vi "FazerGolPelaLateral.vi"(9 "balls":T7[](array[typedef]), 10 "Robot in":T1, 11 "IA State":T6={"our_robots"=[], "enemy_robots"=[], "balls"=[], "geometry"={"field_length"=0, "field_width"=0, "goal_width"=0, "goal_depth"=0, "center_circle_radius"=0, "defense_width"=0, "defense_depth"=0, "free_kick_from_defense_dist"=0, "penalty_spot_from_field_line_dist"=0, "penalty_line_from_spot_dist"=0, "half_moon_depth"=0, "half_moon_width"=0}, "IA Judge"={"stage"="", "command"="", "our_goalie_id"=0.0, "enemy_goalie_id"=0.0, "command enum"=enum."Halt", "Time"=enum."Azul"}, "Received Timestamp"=timestamp(0 s since 1904-01-01), "Events"={"Touch"=FALSE, "id touch"=0.0, "Ball out of \nVision"=FALSE, "Ball inside \nGoalie area"=FALSE, "Robot not responding"=FALSE, "Robots responding status"=[1.0, 1.0, 1.0, 1.0, 1.0, 1.0], "Enemy Ball \nPossession"=FALSE, "Id ini Possession"=0.0, "Ball Possesion"=FALSE, "Id Possesion"=0.0, "Ball at\nour goal side"=FALSE, "Ball at\ntouchline"=FALSE, "Ball at\nenemy goal side"=FALSE}}) -> (3 "Cluster de saída":T1)   [LabVIEW 2018]
doc: "Função que lida com o atacante quando em \"Fazer gol pela lateral\"."
uses:
  Core/AI Robot.ctl
  Intel/Functions Enum.ctl
  Intel/AttackerStates.ctl
  Path Planning/RRT/PathDests.ctl
  Path Planning/RRT/PathDest.ctl
  Core/AI Ball.ctl
  Core/AI Input.ctl
  Core/Field Size.ctl
  Core/AI Judge.ctl
  Intel/Command Enum.ctl
  Util/Events/Events.ctl
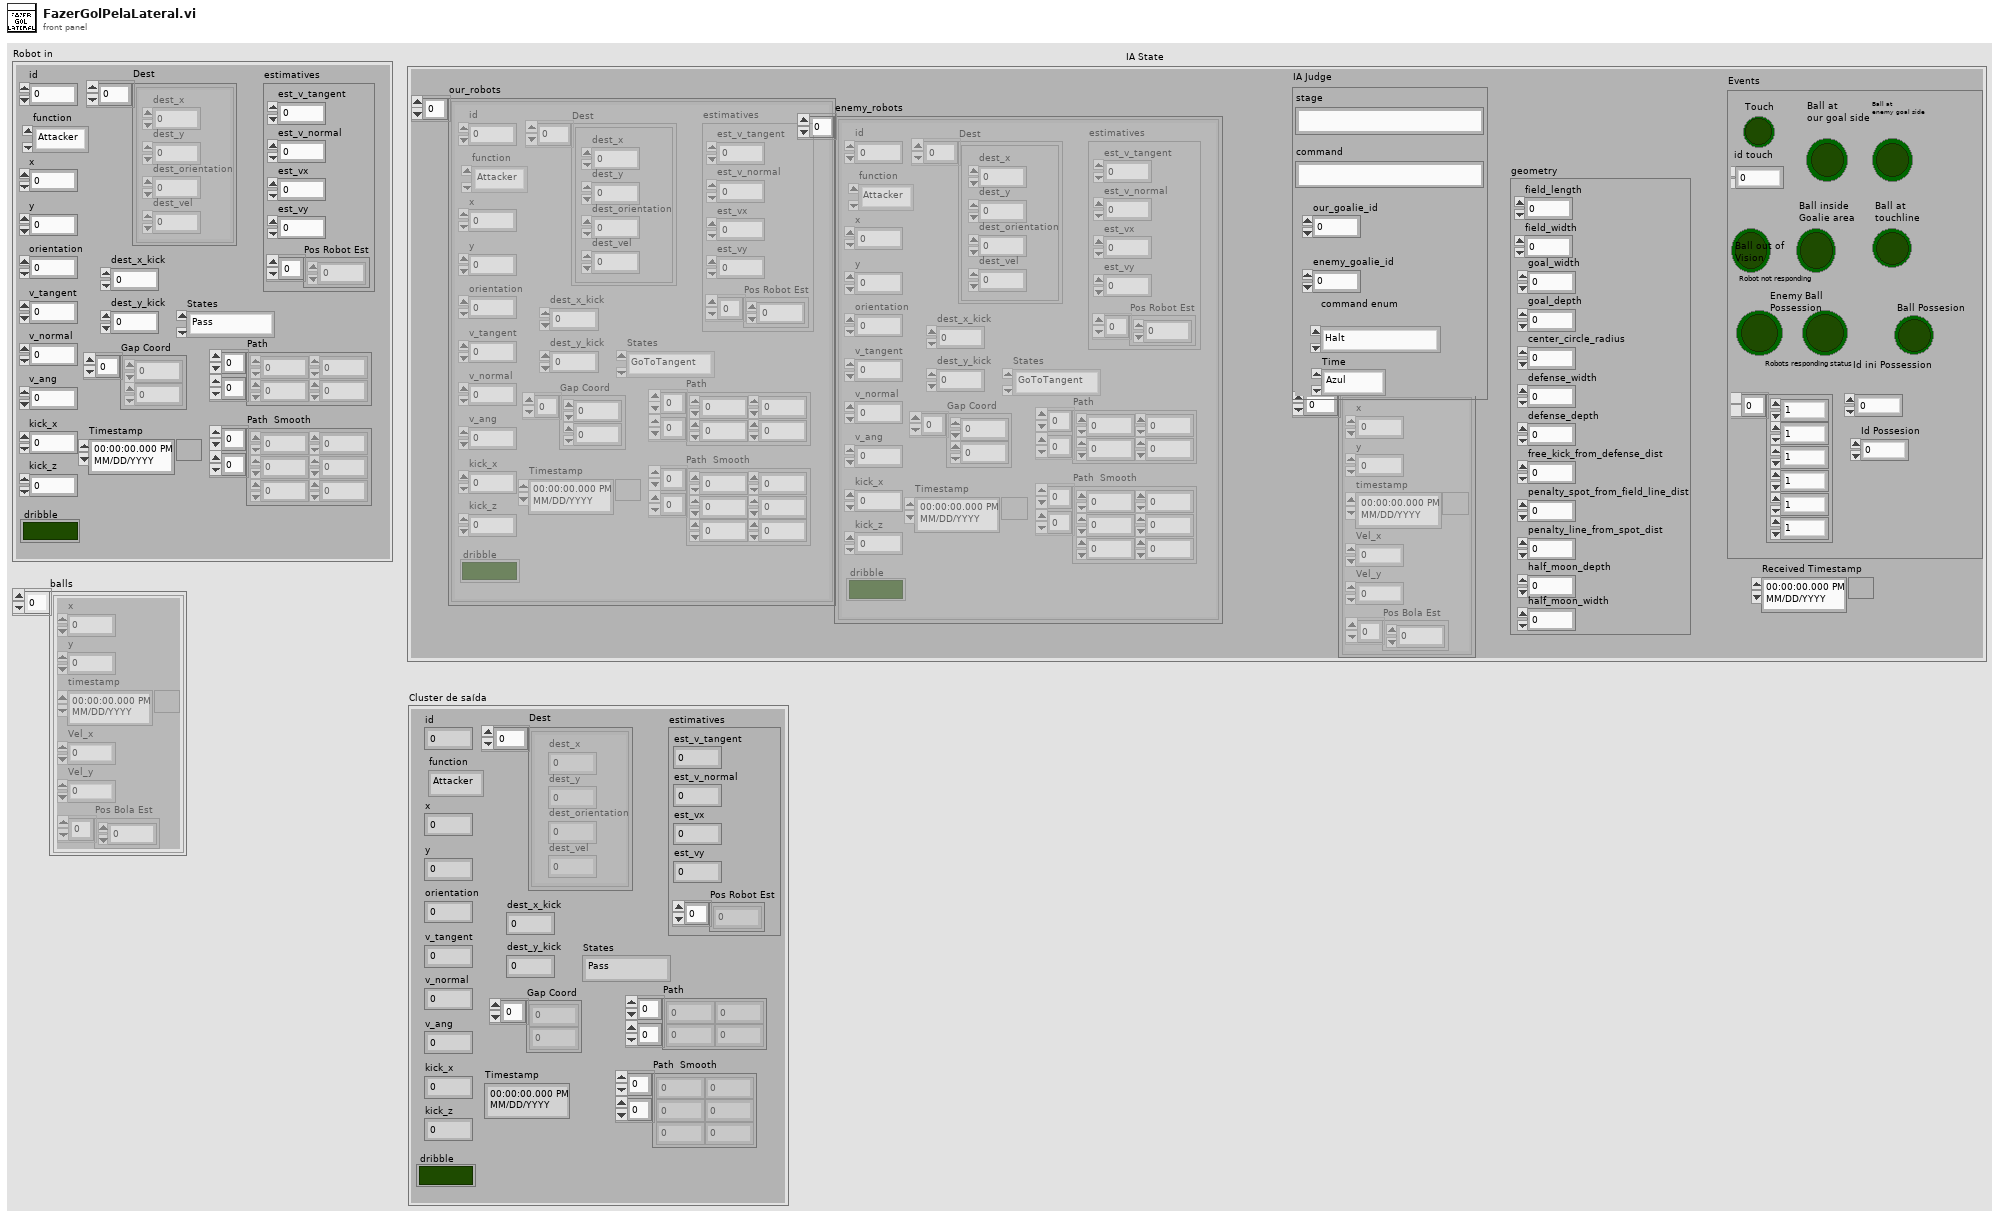
[diagram p1: front panel]
types:
  T1 = typedef "AI Robot.ctl" = cluster{"id":u32, "function":T2, "x":dbl, "y":dbl, "orientation":dbl, "v_tangent":dbl, "v_normal":dbl, "v_ang":dbl, "kick_x":dbl, "kick_z":dbl, "dribble":bool, "Timestamp":timestamp, "estimatives":cluster{"est_v_tangent":dbl, "est_v_normal":dbl, "est_vx":dbl, "est_vy":dbl, "Pos Robot Est":dbl[]}, "dest_x_kick":dbl, "dest_y_kick":dbl, "Gap Coord":dbl[], "States":T3, "Path ":dbl[][], "Path  Smooth":dbl[][], "Dest":T4}
  T2 = typedef "Functions Enum.ctl" = enum16{"Attacker", "Goalie", "Defender", "Striker", "Goto 0", "Dummy", "Kicker", "ZigZag"}
  T3 = typedef "AttackerStates.ctl" = enum16{"Pass", "GoToTangent", "BallGetting", "GoToKick", "Rotate anti-clockwise", "Rotate Clockwise", ""}
  T4 = typedef "PathDests.ctl" = T5[]
  T5 = typedef "PathDest.ctl" = cluster{"dest_x":dbl, "dest_y":dbl, "dest_orientation":dbl, "dest_vel":dbl}
  T6 = typedef "AI Input.ctl" = cluster{"our_robots":T1[], "enemy_robots":T1[], "balls":T7[], "geometry":T8, "IA Judge":T9, "Received Timestamp":timestamp, "Events":T11}
  T7 = typedef "AI Ball.ctl" = cluster{"x":dbl, "y":dbl, "timestamp":timestamp, "Vel_x":dbl, "Vel_y":dbl, "Pos Bola Est":dbl[]}
  T8 = typedef "Field Size.ctl" = cluster{"field_length":u32, "field_width":u32, "goal_width":u32, "goal_depth":u32, "center_circle_radius":u32, "defense_width":u32, "defense_depth":u32, "free_kick_from_defense_dist":u32, "penalty_spot_from_field_line_dist":u32, "penalty_line_from_spot_dist":u32, "half_moon_depth":u32, "half_moon_width":u32}
  T9 = typedef "AI Judge.ctl" = cluster{"stage":string, "command":string, "our_goalie_id":dbl, "enemy_goalie_id":dbl, "command enum":T10, "Time":enum16{"Azul", "Amarelo"}}
  T10 = typedef "Command Enum.ctl" = enum16{"Halt", "Stop", "Force Start", "PKA Normal Start", "Prepare Kickoff Ally", "PKE Normal Start", "Prepare Kickoff Enemy", "Prepare Penalty Ally", "PPA Normal Start", "Prepare Penalty Enemy", "PPE Normal Start", "Ball Placement Enemy Up", "Ball Placement Enemy Down", "Ball Placement Ally Up", "Ball Placement Ally Mid", "Ball Placement Ally Down", "Indirect Free Enemy", "Indirect Free Ally", "Timeout Enemy", "Timeout Ally", "Goal Enemy", "Goal Ally", "Normal Half Time", "Extra Time Break", "Extra Half Time", "None", "Post Game"}
  T11 = typedef "Events.ctl" = cluster{"Touch":bool, "id touch":dbl, "Ball out of \nVision":bool, "Ball inside \nGoalie area":bool, "Robot not responding":bool, "Robots responding status":dbl[], "Enemy Ball \nPossession":bool, "Id ini Possession":dbl, "Ball Possesion":bool, "Id Possesion":dbl, "Ball at\nour goal side":bool, "Ball at\ntouchline":bool, "Ball at\nenemy goal side":bool}
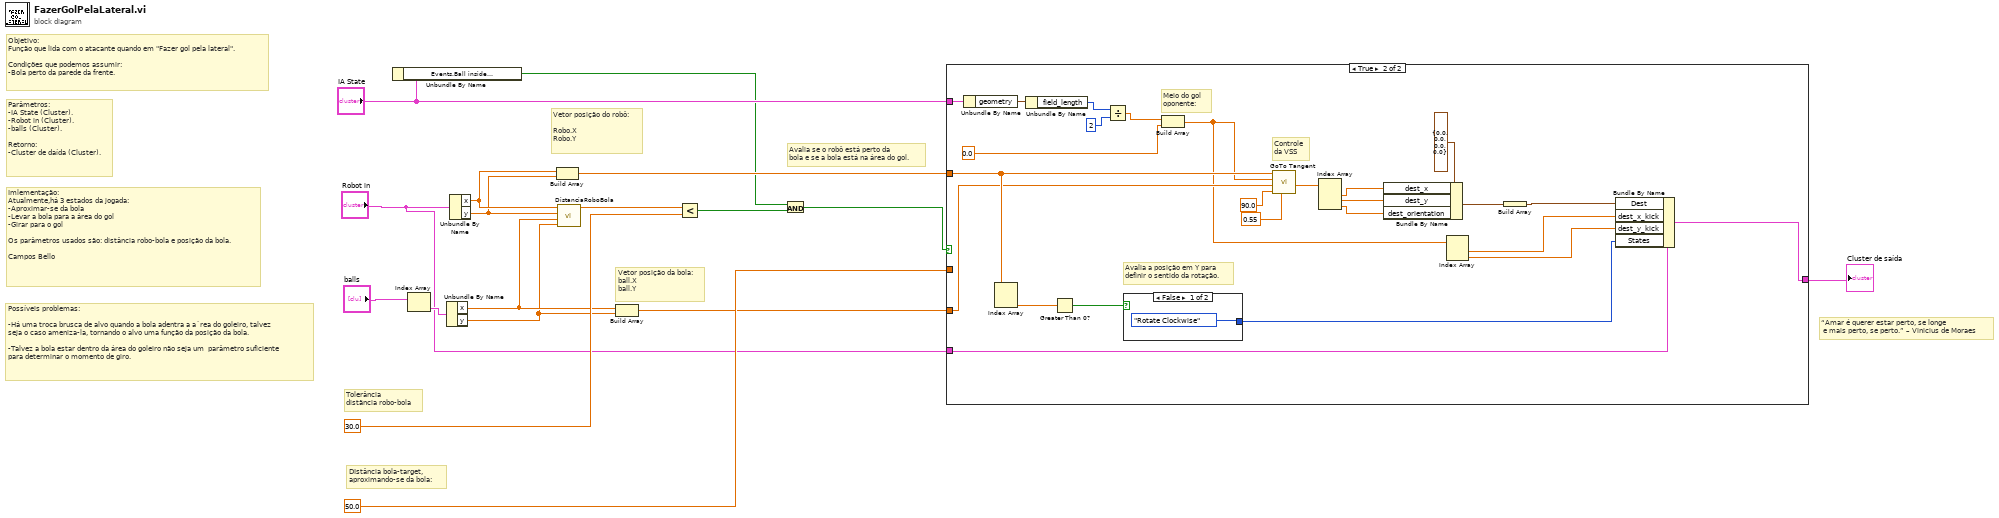
[diagram p0: block diagram]
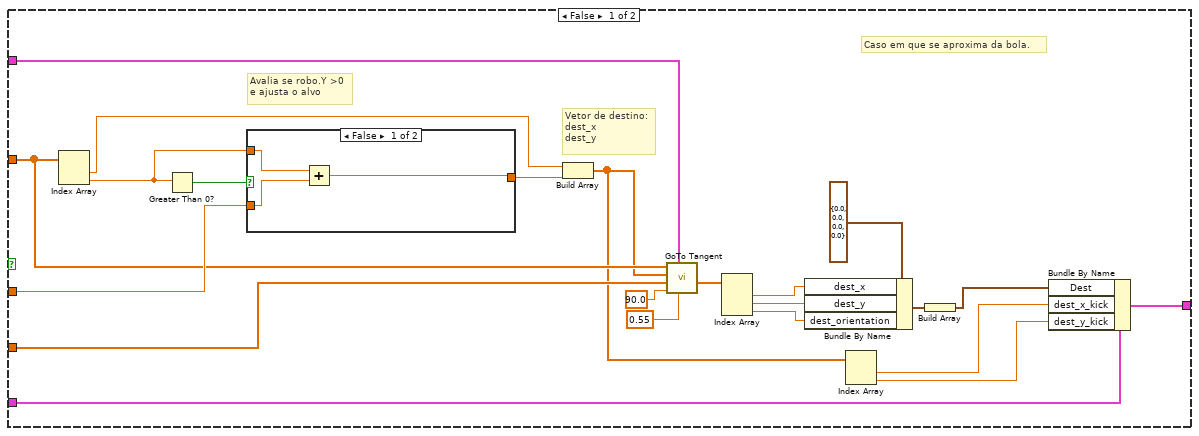
[diagram p2: hidden frame]
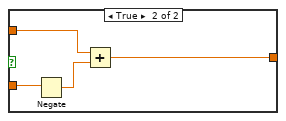
[diagram p3: hidden frame]
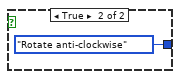
[diagram p4: hidden frame]
diagram:
  # "“Amar é querer estar perto, se longe\n e mais perto, se perto.” – Vinicius de Moraes"
  # "Possíveis problemas:\n\n-Há uma troca brusca de alvo quando a bola adentra a a´rea do goleiro, talvez\nseja o caso ameniza-la, tornando o alvo uma função da posição da bola.\n\n-Talvez a bola estar dentro da área do goleiro não seja um  parâmetro suficiente\npara determinar o momento de giro."
  # "Avalia se o robô está perto da\nbola e se a bola está na área do gol."
  # "Imlementação:\nAtualmente,há 3 estados da jogada:\n-Aproximar-se da bola\n-Levar a bola para a área do gol\n-Girar para o gol\n\nOs parâmetros usados são: distância robo-bola e posição da bola.\n\nCampos Bello"
  # "Parâmetros:\n-IA State (Cluster).\n-Robot in (Cluster).\n-balls (Cluster).\n\nRetorno:\n-Cluster de daída (Cluster)."
  # "Objetivo:\nFunção que lida com o atacante quando em \"Fazer gol pela lateral\".\n\nCondições que podemos assumir:\n-Bola perto da parede da frente."
  # "Vetor posição da bola:\nball.X\nball.Y"
  # "DIstância bola-target,\naproximando-se da bola:"
  # "Vetor posição do robô:\n\nRobo.X\nRobo.Y"
  # "Tolerância\ndistãncia robo-bola"
  n1 = Unbundle By Name("IA State") -> ("Events.Ball inside \nGoalie area"=w3:bool)
  n2 = Index Array(array="balls") -> (element=w16:T7)  [unwired: 1 in]
  n3 = Unbundle By Name(w16) -> ("x"=w9:dbl, "y"=w8:dbl)
  n4 = Unbundle By Name("Robot in") -> ("x"=w13:dbl, "y"=w12:dbl)
  n5 = Build Array(w13, w12) -> (w11:dbl[])
  n6 = call "DistanciaRoboBola.vi"("Y bola"=w8, "X bola"=w9, "Y robo"=w12, "X robo"=w13) -> ("Distância"=w15:dbl)  [unwired: 5 in, 2 out]
  n7 = Build Array(w9, w8) -> (w7:dbl[])
  n8 = Less?(x=w15, y=30.0) -> (x < y?=w4:bool)
  n9 = And(x=w3, y=w4) -> (x .and. y?=w2:bool)
  n10 = case shown="True" w2 {
    tunnel: w11 -> [w32 w63]
    tunnel: 50.0 -> [w36 _]
    tunnel: w7 -> [w31 w62]
    tunnel: "IA State" -> [w30 w71]
    tunnel: "Robot in" -> [w19 w49]
    tunnel: [w18 w47] -> w1
    frame False {
      # "Caso em que se aproxima da bola."
      # "Vetor de destino:\ndest_x\ndest_y"
      # "Avalia se robo.Y >0\ne ajusta o alvo"
      n11 = Index Array(array=w32) -> (element #1=w33:dbl, element #2=w35:dbl)  [unwired: 2 in]
      n12 = Greater Than 0?(x=w35) -> (x > 0?=w37:bool)
      n13 = case shown="False" w37 {
        tunnel: w36 -> [w41 w46]
        tunnel: w35 -> [w42 w45]
        tunnel: [w40 w43] -> w34
        frame False {
          n14 = Add(x=w42, y=w41) -> (x+y=w40:dbl)
        }
        frame True {
          n15 = Negate(x=w46) -> (-x=w44:dbl)
          n16 = Add(x=w45, y=w44) -> (x+y=w43:dbl)
        }
      }
      n17 = Build Array(w33, w34) -> (w22:dbl[])
      n18 = call "GoTo Tangent.vi"("Cone de chute"=0.55, "IA State Input in"=w30, "distance between ball and robot"=90.0, "Ball"=w31, "Target"=w22, "R"=w32) -> ("Destination"=w27:dbl[])  [unwired: 4 in, 1 out]
      n19 = Index Array(array=w27) -> (element #1=w26:dbl, element #2=w25:dbl, element #3=w24:dbl)  [unwired: 3 in]
      n20 = Bundle By Name(cluster=T5 {"dest_x"=0.0, "dest_y"=0.0, "dest_orientation"=0.0, "dest_vel"=0.0} ("element"), "dest_x"=w26, "dest_y"=w25, "dest_orientation"=w24) -> (w28:T5)
      n21 = Index Array(array=w22) -> (element #1=w21:dbl, element #2=w20:dbl)  [unwired: 2 in]
      n22 = Build Array(w28) -> (w23:T5[])
      n23 = Bundle By Name(cluster=w19, "Dest"=w23, "dest_x_kick"=w21, "dest_y_kick"=w20) -> (w18:T1)
    }
    frame True {
      # "Controle\nda VSS"
      # "Avalia a posição em Y para\ndefinir o sentido da rotação."
      # "Meio do gol\noponente:"
      n24 = Unbundle By Name(w71) -> ("geometry"=w70:T8)
      n25 = Index Array(array=w63) -> (element #2=w65:dbl)  [unwired: 2 in, 1 out]
      n26 = Unbundle By Name(w70) -> ("field_length"=w69:u32)
      n27 = Greater Than 0?(x=w65) -> (x > 0?=w64:bool)
      n28 = Divide(x=w69, y=u32 2 ("x")) -> (x/y=w67:dbl)
      n29 = case shown="False" w64 {
        tunnel: [AttackerStates."Rotate Clockwise" ("States") AttackerStates."Rotate anti-clockwise" ("States")] -> w48
        frame False {
        }
        frame True {
        }
      }
      n30 = Build Array(w67, 0.0) -> (w50:dbl[])
      n31 = call "GoTo Tangent.vi"("Cone de chute"=0.55, "distance between ball and robot"=90.0, "Ball"=w62, "Target"=w50, "R"=w63) -> ("Destination"=w54:dbl[])  [unwired: 5 in, 1 out]
      n32 = Index Array(array=w54) -> (element #1=w53:dbl, element #2=w52:dbl, element #3=w51:dbl)  [unwired: 3 in]
      n33 = Bundle By Name(cluster=T5 {"dest_x"=0.0, "dest_y"=0.0, "dest_orientation"=0.0, "dest_vel"=0.0} ("element"), "dest_x"=w53, "dest_y"=w52, "dest_orientation"=w51) -> (w58:T5)
      n34 = Index Array(array=w50) -> (element #1=w56:dbl, element #2=w55:dbl)  [unwired: 2 in]
      n35 = Build Array(w58) -> (w57:T5[])
      n36 = Bundle By Name(cluster=w49, "Dest"=w57, "dest_x_kick"=w56, "dest_y_kick"=w55, "States"=w48) -> (w47:T1)
    }
  }
  "Cluster de saída" <- w1
